vi "TestVI.vi"() -> ()   [LabVIEW 2014]
panel:
  out "Numeric 2":dbl
  in  "Numeric":dbl
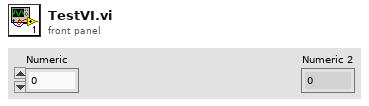
[diagram p1: front panel]
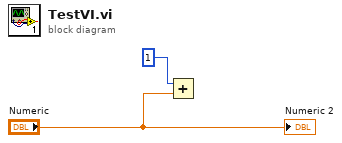
[diagram p0: block diagram]
diagram:
  n1 = Add(x=1, y="Numeric") -> ()  [unwired: 1 out]
  "Numeric 2" <- "Numeric"
